vi "Get APU.vi"(8 "error in (no error)":errorcluster, 11 "APU in":refnum<k24>) -> (0 "error out":errorcluster, 2 "APU Settings":T1 {"des accel" min=0.0 format="%#_p"}, 3 "APU out":refnum<k24>)   [LabVIEW 2020, in "Engine Simulation Toolkit Scripting API.lvlib"]
uses:
  Engine Simulation Toolkit Scripting API.lvlib
  NationalInstruments.VeriStand.SystemDefinitionAPI
  APU Settings.ctl
  Shared/Constants and GUIDs.vi
  Shared/Properties.vi
  <vilib>/NI VeriStand/Custom Device API/Get Item Property (Double).vi
  <vilib>/NI VeriStand/Custom Device Tools/Custom Device Utility Library/NI VeriStand - Search for Item by Name.vi
  <vilib>/NI VeriStand/Custom Device API/Get Item Property (Boolean).vi
  <vilib>/NI VeriStand/Custom Device API/Custom Device API.lvlib
  <vilib>/NI VeriStand/Custom Device Tools/Custom Device Utility Library/Custom Device Utility Library.lvlib
  Shared/Engine Simulation Toolkit Shared.lvlib
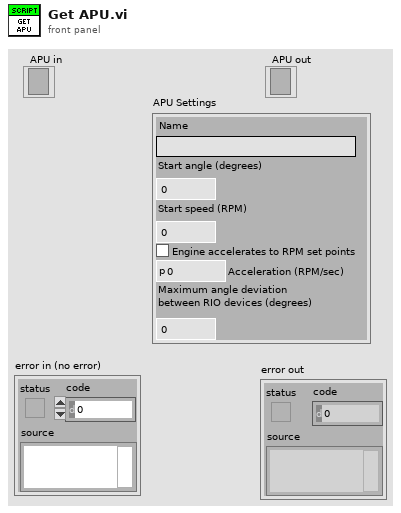
[diagram p1: front panel]
types:
  T1 = typedef "Engine Simulation Toolkit Scripting API.lvlib/APU Settings.ctl" = cluster{"Name":string, "Start angle (degrees)":dbl, "des speed":dbl, "Acceleration":bool, "des accel":dbl, "Maximum angle deviation\nbetween RIO devices (degrees)":dbl}
  T2 = typedef "Engine Simulation Toolkit Shared.lvlib/Channel.ctl" = cluster{"Name":string, "Units":string, "Default":dbl, "Description":string, "Scalable":bool}
  T3 = typedef "Custom Device API.lvlib/Custom Device Item Info.ctl" = cluster{"Name":string, "Is Channel":bool, "GUID":string, "Is Waveform":bool}
  T4 = typedef "Custom Device API.lvlib/Custom Device Item Ref.ctl" = u64
  T5 = typedef "Custom Device API.lvlib/Custom Device Channel.ctl" = cluster{"Type":T6, "Units":string, "Default Value":dbl, "Faultable":bool, "Scalable":bool}
  T6 = typedef "Custom Device API.lvlib/Custom Device Channel Type.ctl" = enum16{"Input", "Output"}
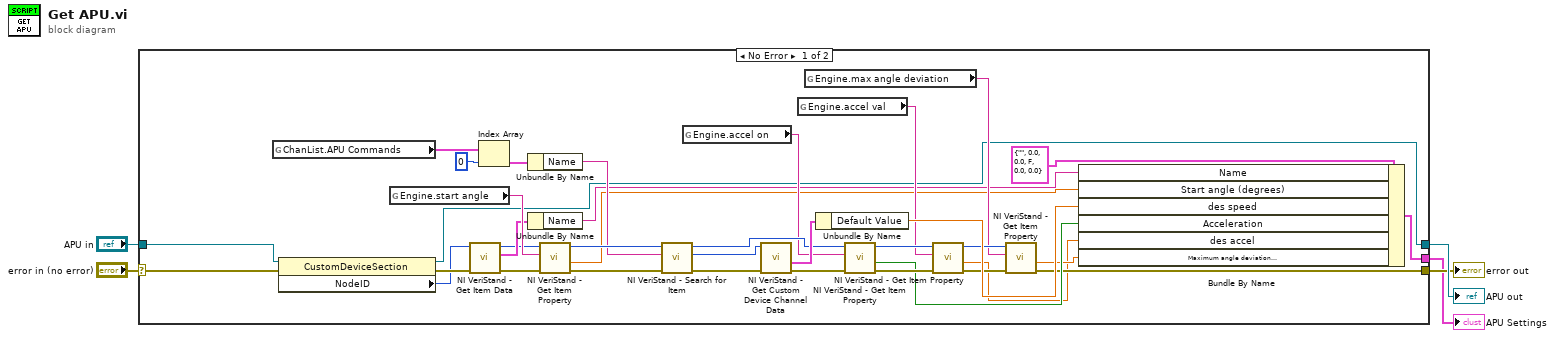
[diagram p0: block diagram]
diagram:
  n1 = case shown="No Error" "error in (no error)" {
    selector: "error in (no error)" -> [w15 w43]
    tunnel: [w17 w43] -> w2
    tunnel: "APU in" -> [w39 w42]
    tunnel: [w16 w42] -> w3
    tunnel: [w40 _] -> w1
    frame No Error {
      n2 = global read "Constants and GUIDs.vi" "ChanList.APU Commands"() -> (w36:T2[])
      n3 = property class="CustomDeviceSection"(reference=w39, error in=w15) -> (reference out=w16:refnum<k24>, error out=w7:errorcluster, "NodeID"=w6:u64)
      n4 = global read "Properties.vi" "Engine.start angle"() -> (w28:string)
      n5 = call <vilib>:"NI VeriStand - Get Item Data.vi"("error in (no error)"=w7, "Item Ref in"=w6) -> ("error out"=w8:errorcluster, "Item Info"=w11:T3, "Item Ref out"=w9:T4)  [unwired: 6 in, 1 out]
      n6 = Index Array(array=w36, index=0) -> (element=w35:T2)
      n7 = Unbundle By Name(w35) -> ("Name"=w33:string)
      n8 = Unbundle By Name(w11) -> ("Name"=w10:string)
      n9 = call-poly <vilib>:"NI VeriStand - Get Item Property.vi"("error in (no error)"=w8, "Property Name"=w28, "Item Ref in"=w9) -> ("error out"=w37:errorcluster, "Value"=w14:dbl, "Item Ref out"=w38:T4)  [unwired: 5 in, 1 out]
      n10 = call-poly <vilib>:"NI VeriStand - Search for Item.vi"("error in"=w37, "Item Name"=w33, "Section Ref in"=w38) -> ("error out"=w30:errorcluster, "Item Ref"=w31:T4, "Section Ref out"=w25:T4)  [unwired: 5 in, 1 out]
      n11 = global read "Properties.vi" "Engine.accel on"() -> (w21:string)
      n12 = call <vilib>:"NI VeriStand - Get Custom Device Channel Data.vi"("error in (no error)"=w30, "Channel Ref in"=w31) -> ("error out"=w24:errorcluster, "Channel"=w32:T5)  [unwired: 4 in, 4 out]
      n13 = global read "Properties.vi" "Engine.accel val"() -> (w19:string)
      n14 = global read "Properties.vi" "Engine.max angle deviation"() -> (w18:string)
      n15 = Unbundle By Name(w32) -> ("Default Value"=w29:dbl)
      n16 = call-poly <vilib>:"NI VeriStand - Get Item Property.vi"("error in (no error)"=w24, "Property Name"=w21, "Item Ref in"=w25) -> ("error out"=w23:errorcluster, "Value"=w20:bool, "Item Ref out"=w26:T4)  [unwired: 5 in, 1 out]
      n17 = call-poly <vilib>:"NI VeriStand - Get Item Property.vi"("error in (no error)"=w23, "Property Name"=w19, "Item Ref in"=w26) -> ("error out"=w22:errorcluster, "Value"=w12:dbl, "Item Ref out"=w27:T4)  [unwired: 5 in, 1 out]
      n18 = call-poly <vilib>:"NI VeriStand - Get Item Property.vi"("error in (no error)"=w22, "Property Name"=w18, "Item Ref in"=w27) -> ("error out"=w17:errorcluster, "Value"=w13:dbl)  [unwired: 5 in, 2 out]
      n19 = Bundle By Name(cluster=T1 {"Name"="", "Start angle (degrees)"=0.0, "des speed"=0.0, "Acceleration"=FALSE, "des accel"=0.0, "Maximum angle deviation\nbetween RIO devices (degrees)"=0.0} ("APU Settings"), "Name"=w10, "Start angle (degrees)"=w14, "des speed"=w29, "Acceleration"=w20, "des accel"=w12, "Maximum angle deviation\nbetween RIO devices (degrees)"=w13) -> (w40:T1)
    }
    frame Error {
    }
  }
  "error out" <- w2
  "APU out" <- w3
  "APU Settings" <- w1
